vi "Process File.vi"(8 "error in (no error)":errorcluster, 10 "File":refnum<class "Acquired Result.lvclass">, 11 "Line Detector in":refnum<class "Line Detector.lvclass">) -> (0 "error out":errorcluster, 2 "File out":refnum<class "Acquired Result.lvclass">, 3 "Line Detector out":refnum<class "Line Detector.lvclass">)   [LabVIEW 2016, in "Line Detector.lvclass"]
uses:
  Line Detector.lvclass
  Results/Acquired Result/Acquired Result.lvclass
  Line Detector.lvclass/Line Detector.ctl
  Results/Acquired Result/Acquired Result.lvclass/Acquired Result.ctl
  Spectrum Recorder too Messages/Update Focus Msg/Update Focus Msg.lvclass
  C:/Program Files (x86)/National Instruments/LabVIEW 2016/vi.lib/ActorFramework/Message/Message.lvclass
  Spectrum Recorder too Messages/Update Focus Msg/Update Focus Msg.lvclass/Update Focus Msg.ctl
  Spectrum Recorder too Messages/Update Focus Msg/Write Focus region centers.vi
  Results/Acquired Result/Write Channels.vi
  Results/Acquired Result/Write Group.vi
  Read Line detector configuration.vi
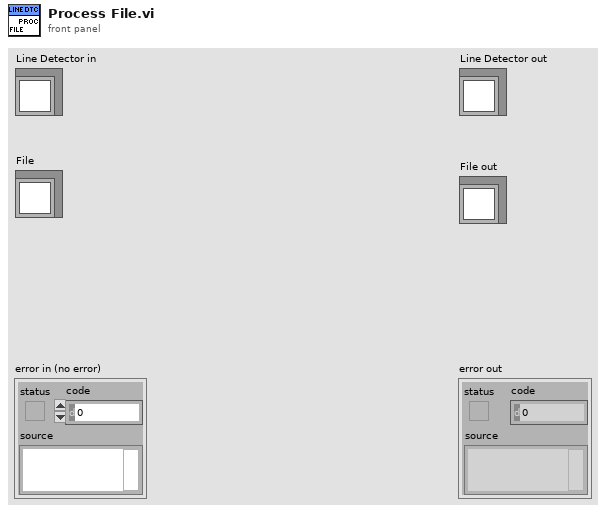
[diagram p1: front panel]
types:
  T1 = enum16{"open", "open or create", "create or replace", "create", "open (read-only)"}
  T2 = typedef "Line Detector Configuration.ctl" = cluster{"Peak width guess":dbl, "Background removal":enum16{"NONE", "High-pass", "Detrend"}, "Smoothing":enum16{"NONE", "Low-pass", "Denoise"}, "Smooth window":dbl, "Relative threshold":dbl, "Finder algorithm":enum16{"Basic", "Wavelet", "Wavelet+detrend"}, "Bgd window":dbl, "Spectrum recorder module name":string, "Fit window":dbl, "Initial fit guess":enum16{"Peak finder", "Last fit"}, "...with header ":string, "Create rusin.dat":bool, "Follow\npeaks":bool, "Re-sample":dbl}
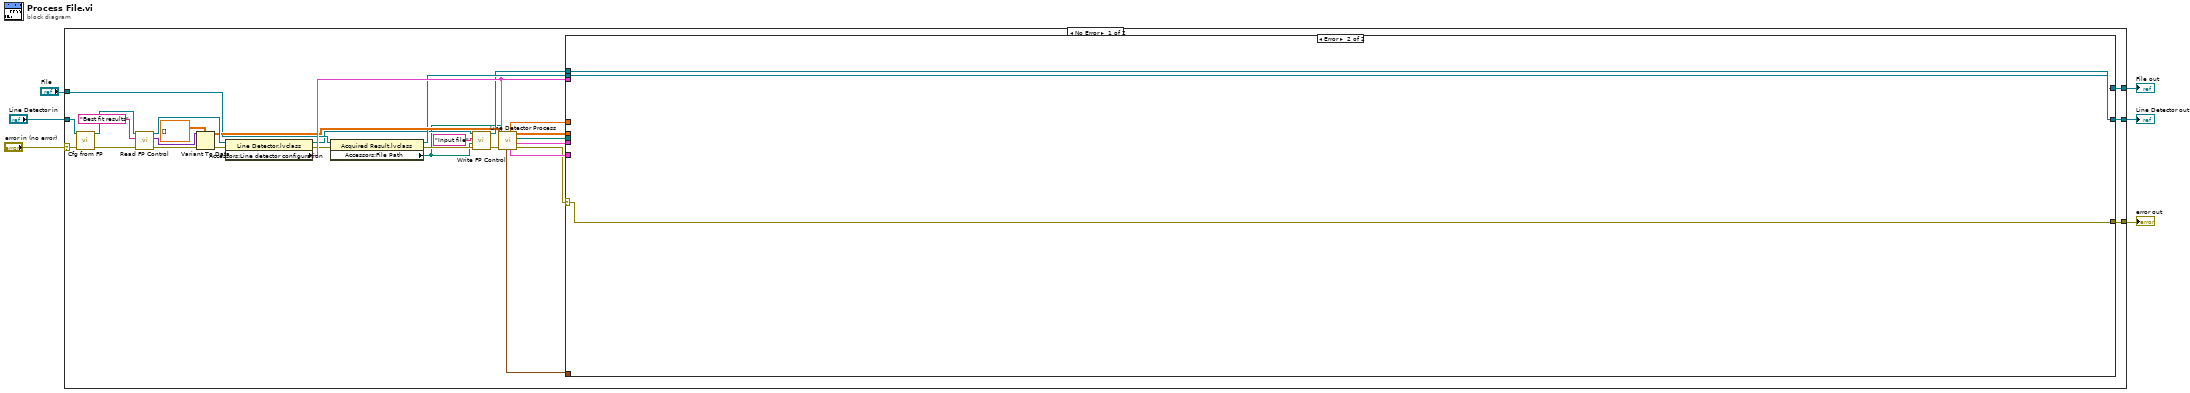
[diagram p0: block diagram]
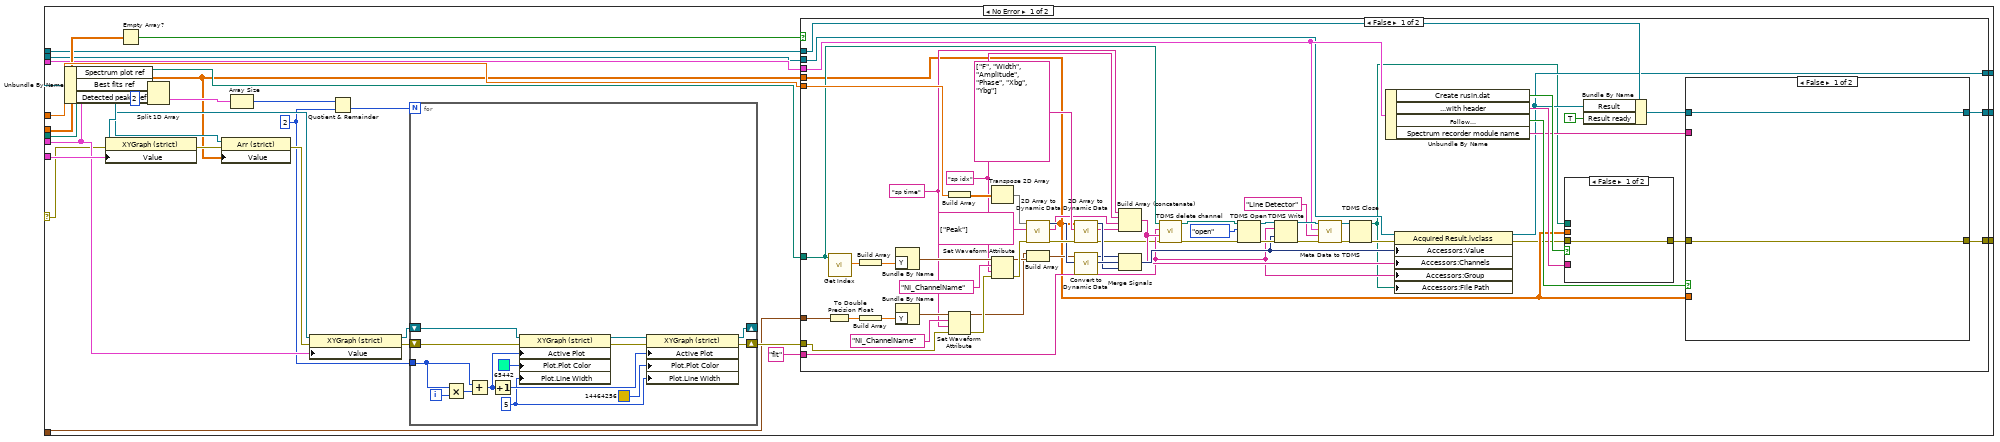
[diagram p2: hidden frame]
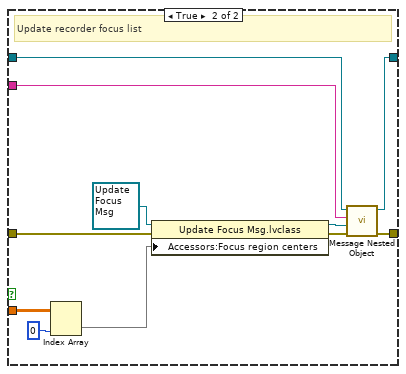
[diagram p3: hidden frame]
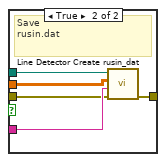
[diagram p4: hidden frame]
diagram:
  n1 = case shown="No Error" "error in (no error)" {
    selector: "error in (no error)" -> [w33 w165]
    tunnel: "Line Detector in" -> [w34 w166]
    tunnel: "File" -> [w17 w167]
    tunnel: [w31 w167] -> w3
    tunnel: [w13 w166] -> w2
    tunnel: [w14 w165] -> w1
    frame No Error {
      n2 = call-dynamic "Cfg from FP.vi"("error in (no error)"=w33, "Measure Object in"=w34) -> ("error out"=w24:errorcluster, "Measure Object out"=w26:refnum<class "Line Detector.lvclass">)  [unwired: 8 in]
      n3 = call-dynamic "Read FP Control.vi"("error in (no error)"=w24, "Control Name"="Best fit results", "Measure Object in"=w26) -> ("error out"=w22:errorcluster, "Control Value"=w21:variant, "Measure Object out"=w25:refnum<class "Line Detector.lvclass">)  [unwired: 5 in, 1 out]
      n4 = Variant To Data(error in=w22, type=dbl[][] [] ("Best fit results"), Variant=w21) -> (data=w18:dbl[][], error out=w20:errorcluster)
      n5 = property class="Line Detector.lvclass"(reference=w25, error in=w20) -> (reference out=w10:refnum<class "Line Detector.lvclass">, error out=w16:errorcluster, "Accessors:Line detector configuration"=w27:T2)
      n6 = property class="Acquired Result.lvclass"(reference=w17, error in=w16) -> (reference out=w15:refnum<class "Acquired Result.lvclass">, error out=w12:errorcluster, "Accessors:File Path"=w7:path)
      n7 = call-dynamic "Write FP Control.vi"("error in (no error)"=w12, "Control Value"=w7, "Control Name"="Input file", "Measure Object in"=w10) -> ("error out"=w11:errorcluster, "Measure Object out"=w9:refnum<class "Line Detector.lvclass">)  [unwired: 6 in]
      n8 = call "Line Detector Process.vi"("error in (no error)"=w11, "Best fit guess"=w18, "File"=w7, "Line Detector Configuration"=w27) -> ("error out"=w8:errorcluster, "Plots"=w36:cluster{"X":dbl[], "Array":dbl[]}[], "File out"=w32:path, "Best fit results"=w29:dbl[][], "Peak Plot"=w37:cluster{"Ramp Pattern":dbl[], "X":dbl[]}[], "Peaks"=w30:dbl[], "sp time"=w28:timestamp)  [unwired: 1 in]
      n9 = case shown="Error" w8 {
        selector: w8 -> [w38 w164]
        tunnel: w37 -> [w64 _]
        tunnel: w36 -> [w58 _]
        tunnel: w32 -> [w51 _]
        tunnel: [w48 w162] -> w31
        tunnel: w30 -> [w46 _]
        tunnel: w29 -> [w45 _]
        tunnel: w28 -> [w44 _]
        tunnel: w27 -> [w43 _]
        tunnel: w15 -> [w42 w162]
        tunnel: [w41 w164] -> w14
        tunnel: [w40 w163] -> w13
        tunnel: w9 -> [w39 w163]
        frame No Error {
          w52 = 2 ("y")
          n10 = Unbundle By Name(w39) -> ("Spectrum plot ref"=w59:refnum<vi>, "Best fits ref"=w63:refnum<vi>, "Detected peaks ref"=w65:refnum<vi>)
          n11 = property class="XYGraph (strict)"(reference=w65, error in=w38, "Value"=w64) -> (error out=w62:errorcluster)  [unwired: 1 out]
          n12 = Empty Array?(array=w45) -> (empty?=w47:bool)
          n13 = Split 1D Array(array=w58, index=2) -> (second subarray=w60:cluster{"X":dbl[], "Array":dbl[]}[])  [unwired: 1 out]
          n14 = property class="Arr (strict)"(reference=w63, error in=w62, "Value"=w45) -> (error out=w57:errorcluster)  [unwired: 1 out]
          n15 = Array Size(array=w60) -> (size(s)=w54:i32)
          n16 = property class="XYGraph (strict)"(reference=w59, error in=w57, "Value"=w58) -> (reference out=w55:refnum<vi>, error out=w56:errorcluster)
          n17 = Quotient & Remainder(x=w54, y=w52) -> (floor(x/y)=w53:i32)  [unwired: 1 out]
          n18 = for {
            N: w53 -> [_]
            shift-right: [w151] -> w50
            shift-left: w56 -> [w160]
            shift-right: [w150] -> _
            shift-left: w55 -> [w161]
            tunnel: w52 -> [w148]
            i -> [w159]
            w152 = u8 5 ("Plot.Line Width")
            n19 = Multiply(x=w148, y=w159) -> (x*y=w149:i32)
            n20 = Add(x=w148, y=w149) -> (x+y=w155:i32)
            n21 = Increment(x=w155) -> (x+1=w154:i32)
            n22 = property class="XYGraph (strict)"(reference=w161, error in=w160, "Active Plot"=w155, "Plot.Plot Color"=u32 65442 ("Color Box"), "Plot.Line Width"=w152) -> (reference out=w157:refnum<vi>, error out=w156:errorcluster)
            n23 = property class="XYGraph (strict)"(reference=w157, error in=w156, "Active Plot"=w154, "Plot.Plot Color"=u32 14464256 ("Color Box"), "Plot.Line Width"=w152) -> (reference out=w150:refnum<vi>, error out=w151:errorcluster)
          }
          n24 = case shown="False" w47 {
            tunnel: w51 -> [w111 _]
            tunnel: w50 -> [w91 w147]
            tunnel: [w77 w147] -> w41
            tunnel: "fit" -> [w100 _]
            tunnel: [w69 w145] -> w48
            tunnel: w46 -> [w118 _]
            tunnel: w45 -> [w74 _]
            tunnel: w39 -> [w99 w146]
            tunnel: [w75 w146] -> w40
            tunnel: w44 -> [w96 _]
            tunnel: w43 -> [w83 _]
            tunnel: w42 -> [w68 w145]
            frame False {
              w88 = "sp time" ("name")
              w102 = "sp idx" ("name")
              n25 = To Double Precision Float(number=w96) -> (double precision float=w90:dbl)
              n26 = call "Get Index.vi"("File Path Control"=w111) -> ("DBL number"=w66:dbl)  [unwired: 9 in, 1 out]
              n27 = Build Array(w66) -> (w110:dbl[])
              n28 = Build Array(w90) -> (w95:dbl[])
              n29 = Bundle By Name("Y"=w110) -> (w109:waveform(dbl))  [unwired: 1 in]
              n30 = Bundle By Name("Y"=w95) -> (w94:waveform(dbl))  [unwired: 1 in]
              n31 = Build Array(w118) -> (w119:dbl[][])
              n32 = Set Waveform Attribute(4:w91, 5:w88, 6:"NI_ChannelName" ("name"), 7:w94) -> (0:w92:errorcluster, 3:w89:waveform(dbl))  [unwired: 1 out]
              n33 = Transpose 2D Array(2D array=w119) -> (transposed array=w97:dbl[][])
              n34 = Set Waveform Attribute(4:w92, 5:w102, 6:"NI_ChannelName" ("name"), 7:w109) -> (0:w107:errorcluster, 3:w106:waveform(dbl))  [unwired: 1 out]
              n35 = call "2D Array to Dynamic Data.vi"("Error In"=w107, "Channels"=string[] ["Peak"], "Array"=w97) -> ("Error Out"=w120:errorcluster, "Channels out"=w113:string[], "Dynamic Data Type"=w117:dynamicdata)  [unwired: 6 in]
              n36 = Build Array(w89, w106) -> (w105:waveform(dbl)[])
              n37 = call "2D Array to Dynamic Data.vi"("Error In"=w120, "Channels"=string[] ["F", "Width", "Amplitude", "Phase", "Xbg", "Ybg"], "Array"=w74) -> ("Error Out"=w72:errorcluster, "Channels out"=w112:string[], "Dynamic Data Type"=w116:dynamicdata)  [unwired: 6 in]
              n38 = call "Convert to Dynamic Data"("Array of Waveforms"=w105) -> ("Dynamic Data Type"=w104:dynamicdata)  [unwired: 3 in]
              n39 = Build Array (concatenate)(w88, w102, w113, w112) -> (w101:string[])
              n40 = Merge Signals(w104, w117, w116) -> (w103:dynamicdata)
              n41 = call "TDMS delete channel.vi"("error in (no error)"=w72, "Channels"=w101, "group name"=w100, "file path"=w111) -> ("error out"=w124:errorcluster, "file path out"=w123:path)  [unwired: 5 in, 1 out]
              n42 = TDMS Open(8:w124, 10:T1."open" ("operation (0:open)"), 11:w123) -> (0:w122:errorcluster, 3:w121:refnum<k34>)  [unwired: 4 in]
              n43 = TDMS Write(0:w121, 5:w100, 9:w103, 11:w122) -> (4:w85:refnum<k34>, 15:w87:errorcluster)  [unwired: 2 in, 2 out]
              n44 = call "Meta Data to TDMS.vi"("Error In"=w87, "Name"="Line Detector", "Value"=w83, "tdms file"=w85) -> ("Error Out"=w86:errorcluster, "tdms file out"=w84:refnum<k34>)  [unwired: 6 in]
              n45 = TDMS Close(8:w86, 11:w84) -> (0:w71:errorcluster, 3:w67:path)
              n46 = Unbundle By Name(w83) -> ("Create rusin.dat"=w82:bool, "...with header"=w81:string, "Follow\npeaks"=w79:bool, "Spectrum recorder module name"=w73:string)
              n47 = property class="Acquired Result.lvclass"(reference=w68, error in=w71, "Accessors:Value"=w103, "Accessors:Channels"=w101, "Accessors:Group"=w100, "Accessors:File Path"=w67) -> (reference out=w69:refnum<class "Acquired Result.lvclass">, error out=w70:errorcluster)
              n48 = case shown="False" w82 {
                tunnel: w81 -> [_ w142]
                tunnel: w67 -> [_ w144]
                tunnel: w74 -> [_ w143]
                tunnel: w70 -> [w139 w141]
                tunnel: [w139 w140] -> w78
                frame False {
                }
                frame True {
                  # "Save\nrusin.dat"
                  n49 = call "Line Detector Create rusin_dat.vi"("Error In"=w141, "header"=w142, "Fit results"=w143, "File Path Control"=w144) -> ("Error Out"=w140:errorcluster)  [unwired: 7 in]
                }
              }
              n50 = Bundle By Name(cluster=w99, "Result"=w69, "Result ready"=TRUE) -> (w76:refnum<class "Line Detector.lvclass">)
              n51 = case shown="False" w79 {
                tunnel: w78 -> [w126 w131]
                tunnel: [w126 w138] -> w77
                tunnel: [w127 w137] -> w75
                tunnel: w76 -> [w127 w136]
                tunnel: w74 -> [_ w135]
                tunnel: w73 -> [_ w133]
                frame False {
                }
                frame True {
                  # "Update recorder focus list"
                  n52 = Index Array(array=w135, index (col)=0 ("index")) -> (element=w130:dbl[])  [unwired: 1 in]
                  n53 = property class="Update Focus Msg.lvclass"(reference=refnum<class "Update Focus Msg.lvclass"> refnum ("Update Focus Msg.lvclass"), error in=w131, "Accessors:Focus region centers"=w130) -> (reference out=w129:refnum<class "Update Focus Msg.lvclass">, error out=w128:errorcluster)
                  n54 = call-dynamic "Message Nested Object.vi"("error in (no error)"=w128, "Message"=w129, "Name"=w133, "Application Controller in"=w136) -> ("error out"=w138:errorcluster, "Application Controller out"=w137:refnum<class "Line Detector.lvclass">)  [unwired: 6 in]
                }
              }
            }
            frame True {
            }
          }
        }
        frame Error {
        }
      }
    }
    frame Error {
    }
  }
  "error out" <- w1
  "Line Detector out" <- w2
  "File out" <- w3
